vi "Computer name.vi"(8 "error in (no error)":errorcluster) -> (0 "error out":errorcluster, 2 "Computer URL":string, 3 "Computer web address":string)   [LabVIEW 2012, in "Design Server.lvlib"]
uses:
  Design Server.lvlib
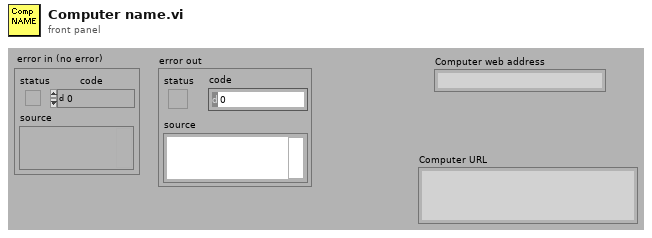
[diagram p1: front panel]
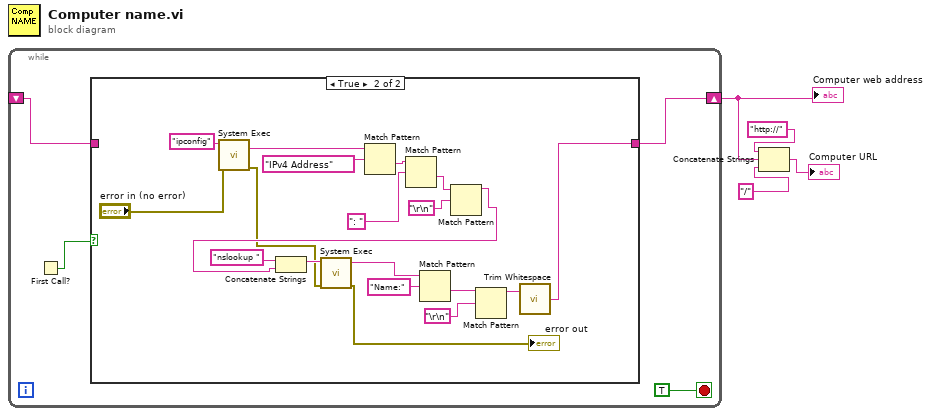
[diagram p0: block diagram]
diagram:
  n1 = while {
    shift-right: [w7] -> w4
    shift-left: _ -> [w6]
    stop <- TRUE stop-if-true
    n2 = First Call?() -> (First Call?: T/F=w5:bool)
    n3 = case shown="True" w5 {
      tunnel: [w9 w10] -> w7
      tunnel: w6 -> [w9 _]
      frame False {
      }
      frame True {
        n4 = call <vilib>:"System Exec.vi"("error in (no error)"="error in (no error)", "command line"="ipconfig") -> ("error out"=w17:errorcluster, "standard output"=w27:string)  [unwired: 6 in, 2 out]
        n5 = Match Pattern(string=w27, regular expression="IPv4 Address") -> (after substring=w25:string)  [unwired: 1 in, 3 out]
        n6 = Match Pattern(string=w25, regular expression=": ") -> (after substring=w22:string)  [unwired: 1 in, 3 out]
        n7 = Match Pattern(string=w22, regular expression="\r\n") -> (before substring=w18:string)  [unwired: 1 in, 3 out]
        n8 = Concatenate Strings("nslookup " ("command line"), w18) -> (w19:string)
        n9 = call <vilib>:"System Exec.vi"("error in (no error)"=w17, "command line"=w19) -> ("error out"=→"error out":errorcluster, "standard output"=w16:string)  [unwired: 6 in, 2 out]
        n10 = Match Pattern(string=w16, regular expression="Name:") -> (after substring=w14:string)  [unwired: 1 in, 3 out]
        n11 = Match Pattern(string=w14, regular expression="\r\n") -> (before substring=w12:string)  [unwired: 1 in, 3 out]
        n12 = call <vilib>:"Trim Whitespace.vi"("string"=w12) -> ("trimmed string"=w10:string)  [unwired: 1 in]
      }
    }
  }
  "Computer web address" <- w4
  n13 = Concatenate Strings("http://", w4, "/") -> (→"Computer URL":string)
